vi "juicer.vi"(8 "error in (no error)":errorcluster, 10 "data":bool[](array[boolean]), 11 "Juicer in":refnum<class "Juicer.lvclass">) -> (0 "error out":errorcluster, 3 "Juicer out":refnum<class "Juicer.lvclass">)   [LabVIEW 2014, in "Juicer.lvclass"]
uses:
  Juicer.lvclass
  Juicer.lvclass/Juicer.ctl
  <vilib>/DAQmx/write.llb/DAQmx Write.vi
  <vilib>/DAQmx/write.llb/DAQmx Write (Digital 1D Bool NChan 1Samp 1Line).vi
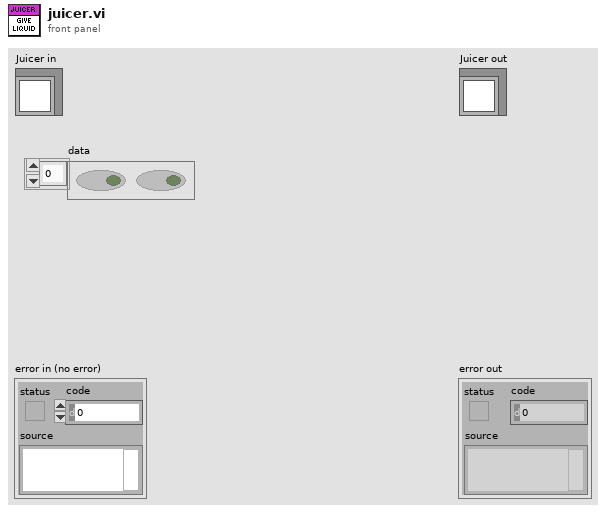
[diagram p1: front panel]
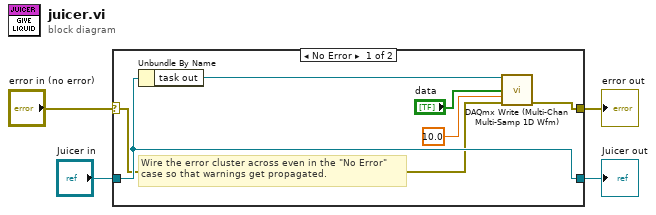
[diagram p0: block diagram]
diagram:
  n1 = case shown="No Error" "error in (no error)" {
    selector: "error in (no error)" -> [w7 w12]
    tunnel: [w6 w12] -> w3
    tunnel: [w9 w11] -> w1
    tunnel: "Juicer in" -> [w9 w11]
    frame No Error {
      # "Wire the error cluster across even in the \"No Error\"\ncase so that warnings get propagated."
      n2 = Unbundle By Name(w9) -> ("task out"=w8:refnum<k21>)
      n3 = call-poly "DAQmx Write (Multi-Chan Multi-Samp 1D Wfm).vi"("task/channels in"=w8, "data"="data", "timeout"=10.0, "error in"=w7) -> ("error out"=w6:errorcluster)  [unwired: 9 in, 2 out]
    }
    frame Error {
    }
  }
  "error out" <- w3
  "Juicer out" <- w1
